vi "Newport ITX-D3N GET Data.vi"(8 "Error In":errorcluster, 11 "TCP Network Connection In":refnum<k5>) -> (0 "Error Out":errorcluster, 1 "Temp/Humidity":dbl[](array[numeric]), 3 "TCP Network Connection Out":refnum<k5>)   [LabVIEW 2016]
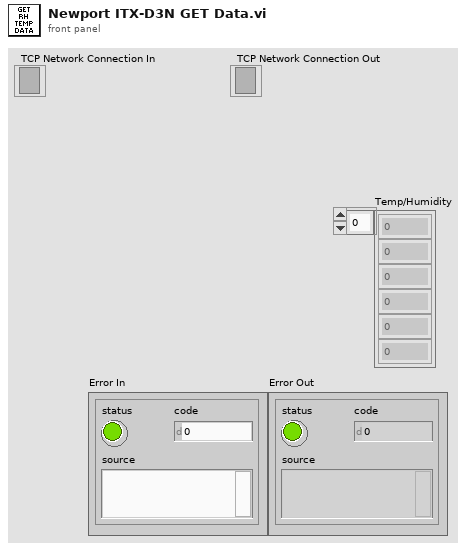
[diagram p1: front panel]
types:
  T1 = enum16{"Standard", "Buffered", "CRLF", "Immediate"}
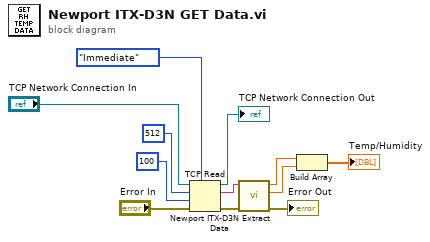
[diagram p0: block diagram]
diagram:
  n1 = TCP Read(connection ID="TCP Network Connection In", bytes to read=512, error in (no error)="Error In", 7:T1."Immediate" ("mode (standard)"), 9:100) -> (connection ID out=→"TCP Network Connection Out":refnum<k5>, data out=w2:string, error out=w4:errorcluster)
  n2 = call "Newport ITX-D3N Extract Data.vi"("Error In"=w4, "TCP String Data"=w2) -> ("Error Out"=→"Error Out":errorcluster, "Relative Humidity"=w5:dbl, "Temperature"=w6:dbl)  [unwired: 6 in, 1 out]
  n3 = Build Array(w6, w5) -> (→"Temp/Humidity":dbl[])
